vi "Settings UI Action.vi"(6 "Mouse Interaction Tag":string, 7 "Action":T1, 11 "UI Data in":refnum<class "Settings UI.lvclass">) -> (3 "UI Data out":refnum<class "Settings UI.lvclass">)   [LabVIEW 2020, in "Output Sequencer.lvlib" / "Settings UI.lvclass"]
uses:
  Settings UI.lvclass
  Types/Settings UI Action.ctl
  Settings UI.lvclass/Settings UI.ctl
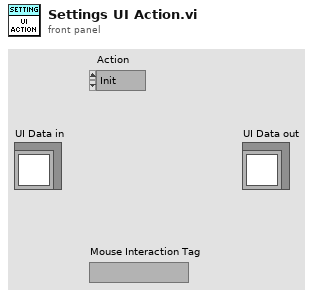
[diagram p1: front panel]
types:
  T1 = typedef "Output Sequencer.lvlib/Settings UI.lvclass/Settings UI Action.ctl" = enum16{"Init", "Timeout", "Tree Change", "Tree Mouse Down/Up", "Value Change", "Expand All", "Show Overview", "Collapse All", "Insert Above", "Insert Below", "Remove Step", "Move Up", "Move Down", "Drag Starting", "Drag Over", "Drop", "Drag Ended", "Import"}
  T2 = typedef "Output Sequencer.lvlib/Settings UI.lvclass/Settings.ctl" = cluster{"Plug-in Version":string, "Step Values":T3[], "Only Execute When Test Running":bool, "Reset Sequence When Test Starts":bool, "Number of Sequence Steps":i32, "Num of Analog Channels":i32, "Num of Digital Channels":i32, "Delay Before Starting Sequence":dbl, "Default Analog Values":dbl[], "Default Digital Values":bool[], "Max Iterations":u32, "Use last value when stopped":bool, "Prioritize exact values":bool, "Enable advanced step timing":bool, "Enable step conditions":bool, "Show confirmation dialogs":bool, "Start condition":string, "Enable re-triggering":bool, "Stop condition":string}
  T3 = typedef "Output Sequencer.lvlib/Settings UI.lvclass/Step Settings.ctl" = cluster{"Description":string, "Precondition":string, "Duration":dbl, "Mode":string, "Delay Between Values":dbl, "Analog Values":string[], "Digital Values":string[], "Postcondition":string, "On True":string, "On False":string}
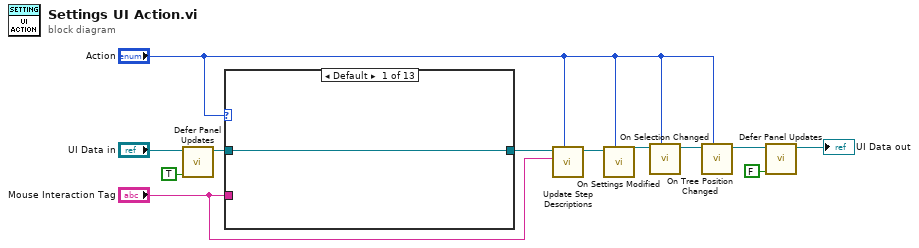
[diagram p0: block diagram]
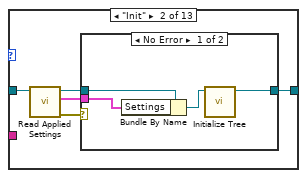
[diagram p2: hidden frame]
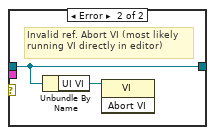
[diagram p3: hidden frame]
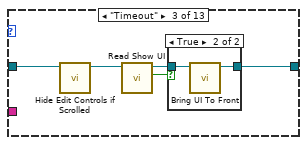
[diagram p4: hidden frame]
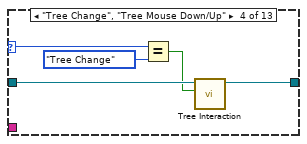
[diagram p6: hidden frame]
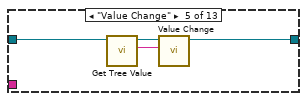
[diagram p7: hidden frame]
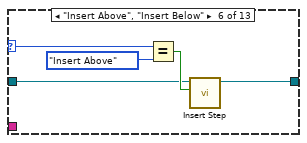
[diagram p8: hidden frame]
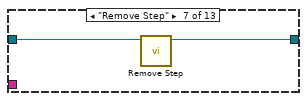
[diagram p9: hidden frame]
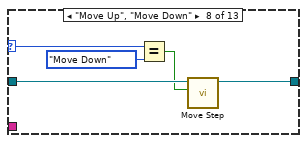
[diagram p10: hidden frame]
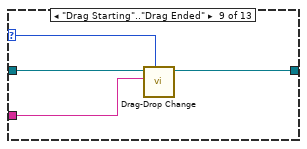
[diagram p11: hidden frame]
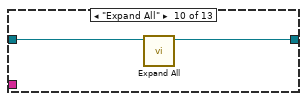
[diagram p12: hidden frame]
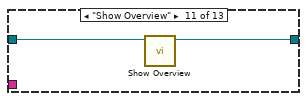
[diagram p13: hidden frame]
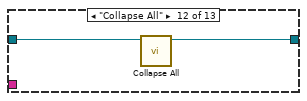
[diagram p14: hidden frame]
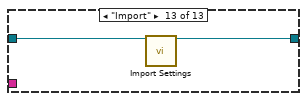
[diagram p15: hidden frame]
diagram:
  n1 = call "Defer Panel Updates.vi"("Defer Panel Updates"=TRUE, "UI Data in"="UI Data in") -> ("UI Data out"=w9:refnum<class "Settings UI.lvclass">)  [unwired: 9 in]
  n2 = case shown="Default" "Action" {
    selector: "Action" -> [_ _ _ w34 _ w46 _ w50 w55 _ _ _ _]
    tunnel: w9 -> [w13 w15 w29 w37 w40 w43 w48 w53 w57 w59 w61 w63 w65]
    tunnel: "Mouse Interaction Tag" -> [_ _ _ _ _ _ _ _ w54 _ _ _ _]
    tunnel: [w13 w18 w25 w36 w38 w42 w47 w52 w56 w58 w60 w62 w64] -> w8
    frame Default {
    }
    frame "Init" {
      n3 = call "Read Applied Settings.vi"("UI Data in"=w15) -> ("error out"=w14:errorcluster, "Applied Settings"=w17:T2, "UI Data out"=w16:refnum<class "Settings UI.lvclass">)  [unwired: 8 in]
      n4 = case shown="No Error" w14 {
        tunnel: [w22 w24] -> w18
        tunnel: w17 -> [w21 _]
        tunnel: w16 -> [w20 w24]
        frame No Error {
          n5 = Bundle By Name(cluster=w20, "Settings"=w21) -> (w19:refnum<class "Settings UI.lvclass">)
          n6 = call "Initialize Tree.vi"("UI Data in"=w19) -> ("UI Data out"=w22:refnum<class "Settings UI.lvclass">)  [unwired: 10 in]
        }
        frame Error {
          # "Invalid ref. Abort VI (most likely\nrunning VI directly in editor)"
          n7 = Unbundle By Name(w24) -> ("UI VI"=w23:refnum<vi>)
          n8 = invoke class="VI" method="Abort VI"(reference=w23) -> ()  [unwired: 2 in, 3 out]
        }
      }
    }
    frame "Timeout" {
      n9 = call "Hide Edit Controls if Scrolled.vi"("Settings UI in"=w29) -> ("Settings UI out"=w27:refnum<class "Settings UI.lvclass">)  [unwired: 10 in]
      n10 = call "Read Show UI.vi"("UI Data in"=w27) -> ("Show UI"=w28:bool, "UI Data out"=w26:refnum<class "Settings UI.lvclass">)  [unwired: 8 in, 1 out]
      n11 = case shown="True" w28 {
        tunnel: w26 -> [w30 w32]
        tunnel: [w30 w31] -> w25
        frame False {
        }
        frame True {
          n12 = call "Bring UI To Front.vi"("UI Data in"=w32) -> ("UI Data out"=w31:refnum<class "Settings UI.lvclass">)  [unwired: 9 in, 1 out]
        }
      }
    }
    frame "Tree Change", "Tree Mouse Down/Up" {
      n13 = Equal?(x=w34, y=Settings_UI_Action."Tree Change" ("Mode")) -> (x = y?=w33:bool)
      n14 = call "Tree Interaction.vi"("Tree Value Changed?"=w33, "Settings UI in"=w37) -> ("Settings UI out"=w36:refnum<class "Settings UI.lvclass">)  [unwired: 9 in]
    }
    frame "Value Change" {
      n15 = call "Get Tree Value.vi"("UI Data in"=w40) -> ("Value"=w39:string, "UI Data out"=w41:refnum<class "Settings UI.lvclass">)  [unwired: 9 in]
      n16 = call "Value Change.vi"("Tree Tag"=w39, "UI Data In"=w41) -> ("UI Data Out"=w38:refnum<class "Settings UI.lvclass">)  [unwired: 9 in]
    }
    frame "Insert Above", "Insert Below" {
      n17 = Equal?(x=w46, y=Settings_UI_Action."Insert Above" ("Mode")) -> (x = y?=w44:bool)
      n18 = call "Insert Step.vi"("Insert Above?"=w44, "Settings UI in"=w43) -> ("Settings UI out"=w42:refnum<class "Settings UI.lvclass">)  [unwired: 9 in]
    }
    frame "Remove Step" {
      n19 = call "Remove Step.vi"("Settings UI in"=w48) -> ("Settings UI out"=w47:refnum<class "Settings UI.lvclass">)  [unwired: 10 in]
    }
    frame "Move Up", "Move Down" {
      n20 = Equal?(x=w50, y=Settings_UI_Action."Move Down") -> (x = y?=w49:bool)
      n21 = call "Move Step.vi"("Move Down?"=w49, "Settings UI in"=w53) -> ("Settings UI out"=w52:refnum<class "Settings UI.lvclass">)  [unwired: 9 in]
    }
    frame "Drag Starting".."Drag Ended" {
      n22 = call "Drag-Drop Change.vi"("Action"=w55, "Mouse Interaction Tag"=w54, "UI Data In"=w57) -> ("UI Data Out"=w56:refnum<class "Settings UI.lvclass">)  [unwired: 8 in]
    }
    frame "Expand All" {
      n23 = call "Expand All.vi"("Settings UI in"=w59) -> ("Settings UI out"=w58:refnum<class "Settings UI.lvclass">)  [unwired: 10 in]
    }
    frame "Show Overview" {
      n24 = call "Show Overview.vi"("UI Data in"=w61) -> ("UI Data out"=w60:refnum<class "Settings UI.lvclass">)  [unwired: 10 in]
    }
    frame "Collapse All" {
      n25 = call "Collapse All.vi"("UI Data in"=w63) -> ("UI Data out"=w62:refnum<class "Settings UI.lvclass">)  [unwired: 10 in]
    }
    frame "Import" {
      n26 = call "Import Settings.vi"("Settings UI in"=w65) -> ("Settings UI out"=w64:refnum<class "Settings UI.lvclass">)  [unwired: 10 in]
    }
  }
  n27 = call "Update Step Descriptions.vi"("Action"="Action", "Mouse Interaction Tag"="Mouse Interaction Tag", "UI Data in"=w8) -> ("UI Data out"=w6:refnum<class "Settings UI.lvclass">)  [unwired: 8 in]
  n28 = call "On Settings Modified.vi"("Action"="Action", "UI Data in"=w6) -> ("UI Data out"=w5:refnum<class "Settings UI.lvclass">)  [unwired: 9 in]
  n29 = call "On Selection Changed.vi"("Action"="Action", "UI Data in"=w5) -> ("UI Data out"=w4:refnum<class "Settings UI.lvclass">)  [unwired: 9 in]
  n30 = call "On Tree Position Changed.vi"("Action"="Action", "Settings UI in"=w4) -> ("Settings UI out"=w3:refnum<class "Settings UI.lvclass">)  [unwired: 9 in]
  n31 = call "Defer Panel Updates.vi"("Defer Panel Updates"=FALSE, "UI Data in"=w3) -> ("UI Data out"=→"UI Data out":refnum<class "Settings UI.lvclass">)  [unwired: 9 in]
